vi "QMH_Dqueue.vi"(6 "timeout in ms (-1)":i32, 8 "error in (no error)":errorcluster, 11 "Queue_ref":refnum<queue>) -> (0 "error out":errorcluster, 2 "Payload":variant, 3 "Message":string)   [LabVIEW 2021, in "Framework_lib.lvlib"]
uses:
  Framework_lib.lvlib
  framework_Qmessage.ctl
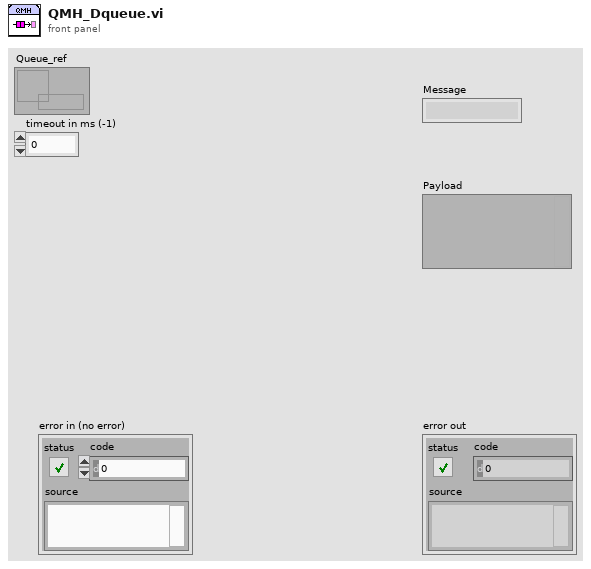
[diagram p1: front panel]
types:
  T1 = typedef "Framework_lib.lvlib/framework_Qmessage.ctl" = cluster{"Message":string, "Payload":variant}
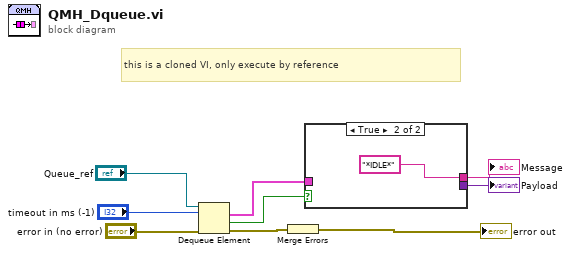
[diagram p0: block diagram]
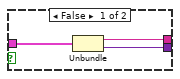
[diagram p2: hidden frame]
diagram:
  # "this is a cloned VI, only execute by reference"
  n1 = Dequeue Element(queue="Queue_ref", timeout in ms (-1)="timeout in ms (-1)", error in (no error)="error in (no error)") -> (element=w7:T1, timed out?=w3:bool, error out=w6:errorcluster)  [unwired: 1 out]
  n2 = Merge Errors(w6) -> (→"error out":errorcluster)
  n3 = case shown="True" w3 {
    tunnel: [w12 _] -> w9
    tunnel: [w11 "*IDLE*" ("Message")] -> w8
    tunnel: w7 -> [w10 _]
    frame False {
      n4 = Unbundle(w10) -> ("Message"=w11:string, "Payload"=w12:variant)
    }
    frame True {
    }
  }
  "Payload" <- w9
  "Message" <- w8
